vi "Binary to LEUI.vi"(7 "Numeric":u8) -> (8 "Blinking Out":T1)   [LabVIEW 2016, in "Centauro.lvlib"]
doc: "This VI converts a binary number to the expected display on LEUI"
uses:
  Projects/Centauro.lvlib
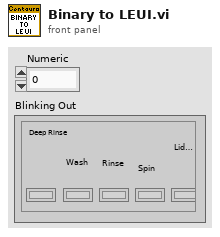
[diagram p1: front panel]
types:
  T1 = cluster{"Deep Rinse":bool, "Wash":bool, "Rinse":bool, "Spin":bool, "Lid Lock":bool}
  T2 = cluster{"[0]":bool, "[1]":bool, "[2]":bool, "[3]":bool, "[4]":bool}
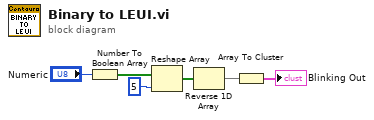
[diagram p0: block diagram]
diagram:
  n1 = Number To Boolean Array(number="Numeric") -> (Boolean array=w5:bool[])
  n2 = Reshape Array(w5, 5 ("dimension size")) -> (w4:bool[])
  n3 = Reverse 1D Array(array=w4) -> (reversed array=w1:bool[])
  n4 = Array To Cluster(array=w1) -> (cluster=→"Blinking Out":T2)
